vi "Test 3.vi"() -> ()   [LabVIEW 2013, in "Generic Data Logger.lvlib" / "Generic Data Logger.lvclass"]
uses:
  Generic Data Logger.lvclass
  <vilib>/Utility/miscctls.llb/LVRectTypeDef.ctl
panel:
  out "i":i32
  in  "y":i16
  out "Front Panel Window:Panel Bounds 2":T1
  out "error out":errorcluster
  in  "Front Panel Window:Panel Bounds":T1
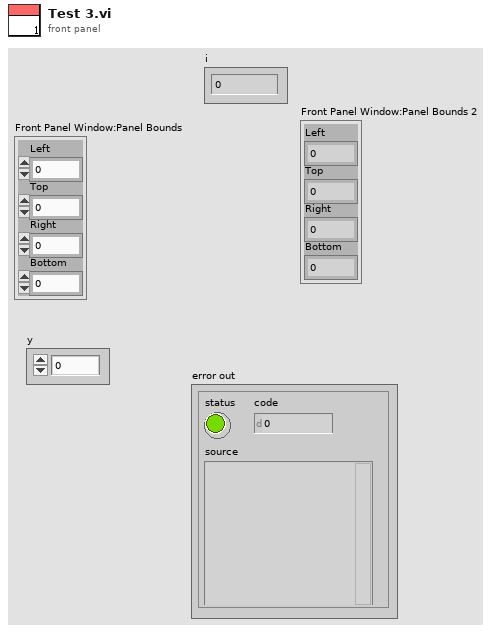
[diagram p1: front panel]
types:
  T1 = typedef "LVRectTypeDef.ctl" = cluster{"Left":i16, "Top":i16, "Right":i16, "Bottom":i16}
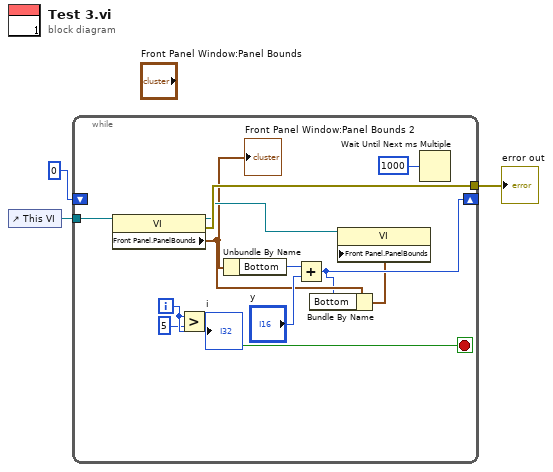
[diagram p0: block diagram]
diagram:
  n1 = control-ref of="This VI"() -> (w2:refnum<vi>)
  n2 = while {
    tunnel: [w15] -> w3
    tunnel: w2 -> [w14]
    shift-right: [w5] -> _
    shift-left: i16 0 ("Bottom") -> [_]
    i -> [w10]
    stop <- w8 stop-if-true
    n3 = property class="VI"(reference=w14) -> (reference out=w7:refnum<vi>, error out=w15:errorcluster, "Front Panel.PanelBounds"=w6:T1)  [unwired: 1 in]
    "Front Panel Window:Panel Bounds 2" <- w6
    n4 = Greater?(x=w10, y=5) -> (0:w8:bool)
    n5 = Unbundle By Name(w6) -> ("Bottom"=w13:i16)
    n6 = Add(x=w13, y="y") -> (x+y=w5:i16)
    n7 = Bundle By Name(cluster=w6, "Bottom"=w5) -> (w4:T1)
    n8 = property class="VI"(reference=w7, "Front Panel.PanelBounds"=w4) -> ()  [unwired: 1 in, 2 out]
    n9 = Wait Until Next ms Multiple(millisecond multiple=u32 1000) -> ()  [unwired: 1 out]
    "i" <- w10
  }
  "error out" <- w3
